vi "Update View.vi"(7 "Team Index":i32, 11 "View":i32[](array[numeric]) caption="View (Team Index, -1: empty)") -> (3 "View out":i32[](array[numeric]) caption="Updated View (-1 team, 0 empty, 1 enemy)")   [LabVIEW 2020, in "DS Square.lvlib"]
uses:
  DS Square.lvlib
panel:
  # "NW\nN\nNE\nE\nSE\nS\nSW\nW"
  # "NW\nN\nNE\nE\nSE\nS\nSW\nW"
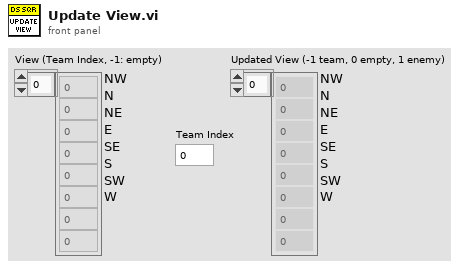
[diagram p1: front panel]
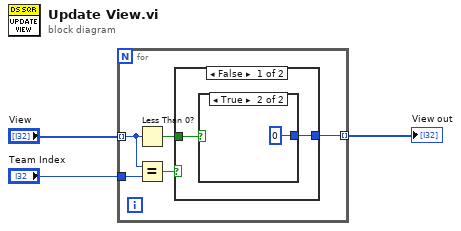
[diagram p0: block diagram]
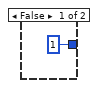
[diagram p2: hidden frame]
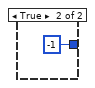
[diagram p3: hidden frame]
diagram:
  n1 = for {
    tunnel: "View" -> [w6] mode=indexing
    tunnel: "Team Index" -> [w8]
    tunnel: [w4] -> w1 mode=indexing
    n2 = Less Than 0?(x=w6) -> (x < 0?=w5:bool)
    n3 = Equal?(x=w6, y=w8) -> (x = y?=w7:bool)
    n4 = case shown="False" w7 {
      tunnel: w5 -> [w10 _]
      tunnel: [w9 -1] -> w4
      frame False {
        n5 = case shown="True" w10 {
          tunnel: [1 0] -> w9
          frame False {
          }
          frame True {
          }
        }
      }
      frame True {
      }
    }
  }
  "View out" <- w1
